vi "frw_device_header.vi"(11 "eeg_device":T1) -> (3 "header array":string[](array[string]))   [LabVIEW 2013]
uses:
  gui/type_def/device.ctl
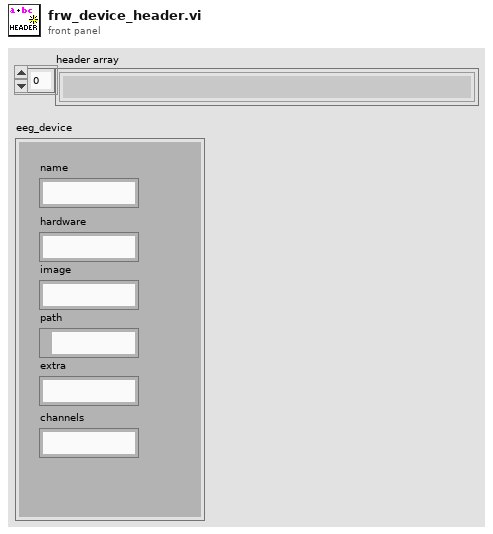
[diagram p1: front panel]
types:
  T1 = typedef "device.ctl" = cluster{"name":string, "hardware":string, "image":string, "path":path, "extra":string, "channels":string}
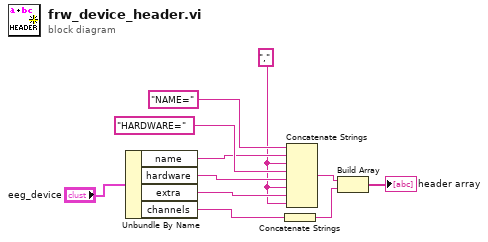
[diagram p0: block diagram]
diagram:
  w1 = "," ("string")
  n1 = Unbundle By Name("eeg_device") -> ("name"=w2:string, "hardware"=w11:string, "extra"=w9:string, "channels"=w8:string)
  n2 = Concatenate Strings(w8) -> (w6:string)
  n3 = Concatenate Strings("NAME=", w2, w1, "HARDWARE=", w11, w1, w9, w1) -> (w7:string)
  n4 = Build Array(w7, w6) -> (→"header array":string[])
